vi "Example.vi"() -> ()   [LabVIEW 2012]
doc: "Example showing operation of the MC Listbox X Control.\nThis VI must be closed to edit the X Control."
uses:
  ListBox_XControl.xctl
panel:
  out "Listbox Value":i32
  in  "Cell Padding (3px)":u32=3
  in  "Column":i32=-1 caption="(-1 = all)"
  in  "Autosize":bool
  in  "stop":bool
  out "ListBox_XControl":i32(xcontrol)
  # "Autosize:"
  # "Example of XControl - This VI must be closed to edit the X Control"
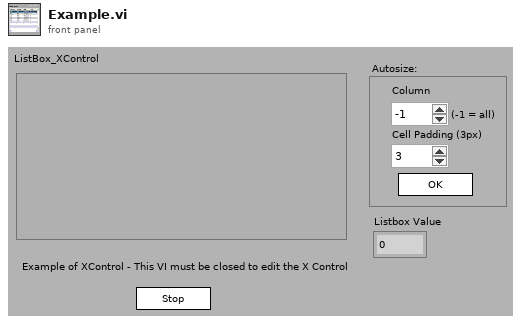
[diagram p1: front panel]
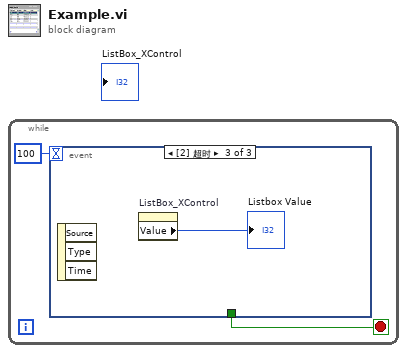
[diagram p0: block diagram]
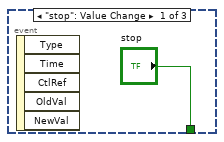
[diagram p2: hidden frame]
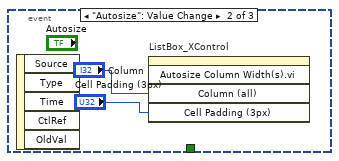
[diagram p3: hidden frame]
diagram:
  n1 = while {
    stop <- w2 stop-if-true
    n2 = event shown="[2] 超时" {
      selector: _ -> [_ _ _]
      dyn-events: _ -> [_ _ _]
      timeout: 100 -> [_ _ _]
      tunnel: ["stop" _ _] -> w2
      event "stop": Value Change {
        n3 = event-data() -> ()  [unwired: 1 in, 5 out]
      }
      event "Autosize": Value Change {
        n4 = event-data() -> ()  [unwired: 1 in, 5 out]
        n5 = invoke on="ListBox_XControl" class="ListBox_XControl (strict)" method="Autosize Column Width(s).vi"("Column (all)"="Column", "Cell Padding (3px)"="Cell Padding (3px)") -> ()  [unwired: 3 in, 5 out]
      }
      event Timeout {
        n6 = event-data() -> ()  [unwired: 1 in, 3 out]
        n7 = property on="ListBox_XControl" class="ListBox_XControl (严格)"() -> ("Value"=→"Listbox Value":i32)  [unwired: 2 in, 2 out]
      }
    }
  }
